vi "XYStage_Load_Command_Array.vi"(8 "error in (no error)":errorcluster, 10 "Command Enumerations":T2(ring), 11 "XY Stage Command Directory":path) -> (0 "error out":errorcluster, 2 "Enumeration Error":bool, 3 "Command Array":T1(array[cluster])=[[{"Serial Command"="ACCEL", "Expected Reply"="null"}, {"Serial Command"="AALIGN", "Expected Reply"=":A"}, {"Serial Command"="AHOME", "Expected Reply"="null"}, {"Serial Command"="AIJ", "Expected Reply"="null"}, {"Serial Command"="ARRAY", "Expected Reply"="null"}, {"Serial Command"="AZERO", "Expected Reply"="null"}, {"Serial Command"="BACKLASH", "Expected Reply"=":A"}, {"Serial Command"="BCUSTOM", "Expected Reply"="null"}, {"Serial Command"="BENABLE", "Expected Reply"="null"}, {"Serial Command"="BUILD", "Expected Reply"="null"}, {"Serial Command"="CDATE", "Expected Reply"="null"}, {"Serial Command"="CNTS", "Expected Reply"=":A"}, {"Serial Command"="CUSTOMA", "Expected Reply"="null"}, {"Serial Command"="CUSTOMB", "Expected Reply"="null"}, {"Serial Command"="DACK", "Expected Reply"=":A"}, {"Serial Command"="DUMP", "Expected Reply"="null"}, {"Serial Command"="ENSYNC", "Expected Reply"="null"}, {"Serial Command"="EPOLARITY", "Expected Reply"="null"}, {"Serial Command"="ERROR", "Expected Reply"=":A"}, {"Serial Command"="HALT", "Expected Reply"=":A"}, {"Serial Command"="HERE", "Expected Reply"=":A"}, {"Serial Command"="HOME", "Expected Reply"=":A"}, {"Serial Command"="INFO", "Expected Reply"="Ax"}, {"Serial Command"="JOYSTICK", "Expected Reply"=":A"}, {"Serial Command"="JSSPD", "Expected Reply"=":A"}, {"Serial Command"="KD", "Expected Reply"="null"}, {"Serial Command"="KI", "Expected Reply"="null"}, {"Serial Command"="KP", "Expected Reply"="null"}, {"Serial Command"="LCD", "Expected Reply"="null"}, {"Serial Command"="LED", "Expected Reply"="null"}, {"Serial Command"="LLADDR", "Expected Reply"="null"}, {"Serial Command"="LOAD", "Expected Reply"="null"}, {"Serial Command"="MAINTAIN", "Expected Reply"=":A"}, {"Serial Command"="MOTCTRL", "Expected Reply"=":A"}, {"Serial Command"="MOVE", "Expected Reply"=":A"}, {"Serial Command"="MOVREL", "Expected Reply"=":A"}, {"Serial Command"="PCROS", "Expected Reply"=":A"}, {"Serial Command"="PEDAL", "Expected Reply"=":A"}, {"Serial Command"="RBMODE", "Expected Reply"="null"}, {"Serial Command"="RDADC", "Expected Reply"=":A"}, {"Serial Command"="RDSBYTE", "Expected Reply"="null"}, {"Serial Command"="RDSTAT", "Expected Reply"=":A"}, {"Serial Command"="RESET", "Expected Reply"=":A"}, {"Serial Command"="RT", "Expected Reply"=":A"}, {"Serial Command"="RUNAWAY", "Expected Reply"=":A"}, {"Serial Command"="SAVESET", "Expected Reply"=":A"}, {"Serial Command"="SAVEPOS", "Expected Reply"=":A"}, {"Serial Command"="SCAN", "Expected Reply"="null"}, {"Serial Command"="SCANR", "Expected Reply"="null"}, {"Serial Command"="SCANV", "Expected Reply"="null"}, {"Serial Command"="SECURE", "Expected Reply"=":A"}, {"Serial Command"="SETHOME", "Expected Reply"=":A"}, {"Serial Command"="SETLOW", "Expected Reply"=":A"}, {"Serial Command"="SETUP", "Expected Reply"="null"}, {"Serial Command"="SI", "Expected Reply"=":A"}, {"Serial Command"="SPEED", "Expected Reply"=":A"}, {"Serial Command"="SPIN", "Expected Reply"=":A"}, {"Serial Command"="STATUS", "Expected Reply"="N"}, {"Serial Command"="STOPBITS", "Expected Reply"="null"}, {"Serial Command"="TTL", "Expected Reply"="null"}, {"Serial Command"="UM", "Expected Reply"=":A"}, {"Serial Command"="UNITS", "Expected Reply"=":A"}, {"Serial Command"="VB", "Expected Reply"="null"}, {"Serial Command"="VECTOR", "Expected Reply"=":A"}, {"Serial Command"="VERSION", "Expected Reply"=":A"}, {"Serial Command"="WAIT", "Expected Reply"=":A"}, {"Serial Command"="WHERE", "Expected Reply"=":A"}, {"Serial Command"="WHO", "Expected Reply"=":A"}, {"Serial Command"="WRDAC", "Expected Reply"=":A"}, {"Serial Command"="ZERO", "Expected Reply"=":A"}, {"Serial Command"="Z2B", "Expected Reply"=":A"}, {"Serial Command"="ZS", "Expected Reply"=":A"}, {"Serial Command"="OPEN", "Expected Reply"="null"}, {"Serial Command"="CLOSE", "Expected Reply"="null"}, {"Serial Command"="-0.1", "Expected Reply"="null"}, {"Serial Command"="0.1", "Expected Reply"="null"}, {"Serial Command"="75000", "Expected Reply"="null"}], [{"Serial Command"="ACCEL", "Expected Reply"="null"}, {"Serial Command"="AALIGN", "Expected Reply"=":A"}, {"Serial Command"="AHOME", "Expected Reply"="null"}, {"Serial Command"="AIJ", "Expected Reply"="null"}, {"Serial Command"="ARRAY", "Expected Reply"="null"}, {"Serial Command"="AZERO", "Expected Reply"="null"}, {"Serial Command"="BACKLASH", "Expected Reply"=":A"}, {"Serial Command"="BCUSTOM", "Expected Reply"="null"}, {"Serial Command"="BENABLE", "Expected Reply"="null"}, {"Serial Command"="BUILD", "Expected Reply"="null"}, {"Serial Command"="CDATE", "Expected Reply"="null"}, {"Serial Command"="CNTS", "Expected Reply"=":A"}, {"Serial Command"="CUSTOMA", "Expected Reply"="null"}, {"Serial Command"="CUSTOMB", "Expected Reply"="null"}, {"Serial Command"="DACK", "Expected Reply"=":A"}, {"Serial Command"="DUMP", "Expected Reply"="null"}, {"Serial Command"="ENSYNC", "Expected Reply"="null"}, {"Serial Command"="EPOLARITY", "Expected Reply"="null"}, {"Serial Command"="ERROR", "Expected Reply"=":A"}, {"Serial Command"="HALT", "Expected Reply"=":A"}, {"Serial Command"="HERE", "Expected Reply"=":A"}, {"Serial Command"="HOME", "Expected Reply"=":A"}, {"Serial Command"="INFO", "Expected Reply"="Ax"}, {"Serial Command"="JOYSTICK", "Expected Reply"=":A"}, {"Serial Command"="JSSPD", "Expected Reply"=":A"}, {"Serial Command"="KD", "Expected Reply"="null"}, {"Serial Command"="KI", "Expected Reply"="null"}, {"Serial Command"="KP", "Expected Reply"="null"}, {"Serial Command"="LCD", "Expected Reply"="null"}, {"Serial Command"="LED", "Expected Reply"="null"}, {"Serial Command"="LLADDR", "Expected Reply"="null"}, {"Serial Command"="LOAD", "Expected Reply"="null"}, {"Serial Command"="MAINTAIN", "Expected Reply"=":A"}, {"Serial Command"="MOTCTRL", "Expected Reply"=":A"}, {"Serial Command"="MOVE", "Expected Reply"=":A"}, {"Serial Command"="MOVREL", "Expected Reply"=":A"}, {"Serial Command"="PCROS", "Expected Reply"=":A"}, {"Serial Command"="PEDAL", "Expected Reply"=":A"}, {"Serial Command"="RBMODE", "Expected Reply"="null"}, {"Serial Command"="RDADC", "Expected Reply"=":A"}, {"Serial Command"="RDSBYTE", "Expected Reply"="null"}, {"Serial Command"="RDSTAT", "Expected Reply"=":A"}, {"Serial Command"="RESET", "Expected Reply"=":A"}, {"Serial Command"="RT", "Expected Reply"=":A"}, {"Serial Command"="RUNAWAY", "Expected Reply"=":A"}, {"Serial Command"="SAVESET", "Expected Reply"=":A"}, {"Serial Command"="SAVEPOS", "Expected Reply"=":A"}, {"Serial Command"="SCAN", "Expected Reply"="null"}, {"Serial Command"="SCANR", "Expected Reply"="null"}, {"Serial Command"="SCANV", "Expected Reply"="null"}, {"Serial Command"="SECURE", "Expected Reply"=":A"}, {"Serial Command"="SETHOME", "Expected Reply"=":A"}, {"Serial Command"="SETLOW", "Expected Reply"=":A"}, {"Serial Command"="SETUP", "Expected Reply"="null"}, {"Serial Command"="SI", "Expected Reply"=":A"}, {"Serial Command"="SPEED", "Expected Reply"=":A"}, {"Serial Command"="SPIN", "Expected Reply"=":A"}, {"Serial Command"="STATUS", "Expected Reply"="N"}, {"Serial Command"="STOPBITS", "Expected Reply"="null"}, {"Serial Command"="TTL", "Expected Reply"="null"}, {"Serial Command"="UM", "Expected Reply"=":A"}, {"Serial Command"="UNITS", "Expected Reply"=":A"}, {"Serial Command"="VB", "Expected Reply"="null"}, {"Serial Command"="VECTOR", "Expected Reply"=":A"}, {"Serial Command"="VERSION", "Expected Reply"=":A"}, {"Serial Command"="WAIT", "Expected Reply"=":A"}, {"Serial Command"="WHERE", "Expected Reply"=":A"}, {"Serial Command"="WHO", "Expected Reply"=":A"}, {"Serial Command"="WRDAC", "Expected Reply"=":A"}, {"Serial Command"="ZERO", "Expected Reply"=":A"}, {"Serial Command"="Z2B", "Expected Reply"=":A"}, {"Serial Command"="ZS", "Expected Reply"=":A"}, {"Serial Command"="OPEN", "Expected Reply"="null"}, {"Serial Command"="CLOSE", "Expected Reply"="null"}, {"Serial Command"="-0.1", "Expected Reply"="null"}, {"Serial Command"="0.1", "Expected Reply"="null"}, {"Serial Command"="75000", "Expected Reply"="null"}], [{"Serial Command"="ACCEL", "Expected Reply"="null"}, {"Serial Command"="AALIGN", "Expected Reply"=":A"}, {"Serial Command"="AHOME", "Expected Reply"="null"}, {"Serial Command"="AIJ", "Expected Reply"="null"}, {"Serial Command"="ARRAY", "Expected Reply"="null"}, {"Serial Command"="AZERO", "Expected Reply"="null"}, {"Serial Command"="BACKLASH", "Expected Reply"=":A"}, {"Serial Command"="BCUSTOM", "Expected Reply"="null"}, {"Serial Command"="BENABLE", "Expected Reply"="null"}, {"Serial Command"="BUILD", "Expected Reply"="null"}, {"Serial Command"="CDATE", "Expected Reply"="null"}, {"Serial Command"="CNTS", "Expected Reply"=":A"}, {"Serial Command"="CUSTOMA", "Expected Reply"="null"}, {"Serial Command"="CUSTOMB", "Expected Reply"="null"}, {"Serial Command"="DACK", "Expected Reply"=":A"}, {"Serial Command"="DUMP", "Expected Reply"="null"}, {"Serial Command"="ENSYNC", "Expected Reply"="null"}, {"Serial Command"="EPOLARITY", "Expected Reply"="null"}, {"Serial Command"="ERROR", "Expected Reply"=":A"}, {"Serial Command"="HALT", "Expected Reply"=":A"}, {"Serial Command"="HERE", "Expected Reply"=":A"}, {"Serial Command"="HOME", "Expected Reply"=":A"}, {"Serial Command"="INFO", "Expected Reply"="Ax"}, {"Serial Command"="JOYSTICK", "Expected Reply"=":A"}, {"Serial Command"="JSSPD", "Expected Reply"=":A"}, {"Serial Command"="KD", "Expected Reply"="null"}, {"Serial Command"="KI", "Expected Reply"="null"}, {"Serial Command"="KP", "Expected Reply"="null"}, {"Serial Command"="LCD", "Expected Reply"="null"}, {"Serial Command"="LED", "Expected Reply"="null"}, {"Serial Command"="LLADDR", "Expected Reply"="null"}, {"Serial Command"="LOAD", "Expected Reply"="null"}, {"Serial Command"="MAINTAIN", "Expected Reply"=":A"}, {"Serial Command"="MOTCTRL", "Expected Reply"=":A"}, {"Serial Command"="MOVE", "Expected Reply"=":A"}, {"Serial Command"="MOVREL", "Expected Reply"=":A"}, {"Serial Command"="PCROS", "Expected Reply"=":A"}, {"Serial Command"="PEDAL", "Expected Reply"=":A"}, {"Serial Command"="RBMODE", "Expected Reply"="null"}, {"Serial Command"="RDADC", "Expected Reply"=":A"}, {"Serial Command"="RDSBYTE", "Expected Reply"="null"}, {"Serial Command"="RDSTAT", "Expected Reply"=":A"}, {"Serial Command"="RESET", "Expected Reply"=":A"}, {"Serial Command"="RT", "Expected Reply"=":A"}, {"Serial Command"="RUNAWAY", "Expected Reply"=":A"}, {"Serial Command"="SAVESET", "Expected Reply"=":A"}, {"Serial Command"="SAVEPOS", "Expected Reply"=":A"}, {"Serial Command"="SCAN", "Expected Reply"="null"}, {"Serial Command"="SCANR", "Expected Reply"="null"}, {"Serial Command"="SCANV", "Expected Reply"="null"}, {"Serial Command"="SECURE", "Expected Reply"=":A"}, {"Serial Command"="SETHOME", "Expected Reply"=":A"}, {"Serial Command"="SETLOW", "Expected Reply"=":A"}, {"Serial Command"="SETUP", "Expected Reply"="null"}, {"Serial Command"="SI", "Expected Reply"=":A"}, {"Serial Command"="SPEED", "Expected Reply"=":A"}, {"Serial Command"="SPIN", "Expected Reply"=":A"}, {"Serial Command"="STATUS", "Expected Reply"="N"}, {"Serial Command"="STOPBITS", "Expected Reply"="null"}, {"Serial Command"="TTL", "Expected Reply"="null"}, {"Serial Command"="UM", "Expected Reply"=":A"}, {"Serial Command"="UNITS", "Expected Reply"=":A"}, {"Serial Command"="VB", "Expected Reply"="null"}, {"Serial Command"="VECTOR", "Expected Reply"=":A"}, {"Serial Command"="VERSION", "Expected Reply"=":A"}, {"Serial Command"="WAIT", "Expected Reply"=":A"}, {"Serial Command"="WHERE", "Expected Reply"=":A"}, {"Serial Command"="WHO", "Expected Reply"=":A"}, {"Serial Command"="WRDAC", "Expected Reply"=":A"}, {"Serial Command"="ZERO", "Expected Reply"=":A"}, {"Serial Command"="Z2B", "Expected Reply"=":A"}, {"Serial Command"="ZS", "Expected Reply"=":A"}, {"Serial Command"="OPEN", "Expected Reply"="null"}, {"Serial Command"="CLOSE", "Expected Reply"="null"}, {"Serial Command"="-0.1", "Expected Reply"="null"}, {"Serial Command"="0.1", "Expected Reply"="null"}, {"Serial Command"="75000", "Expected Reply"="null"}]])   [LabVIEW 2013]
uses:
  <vilib>/Utility/file.llb/Read From Spreadsheet File (string).vi
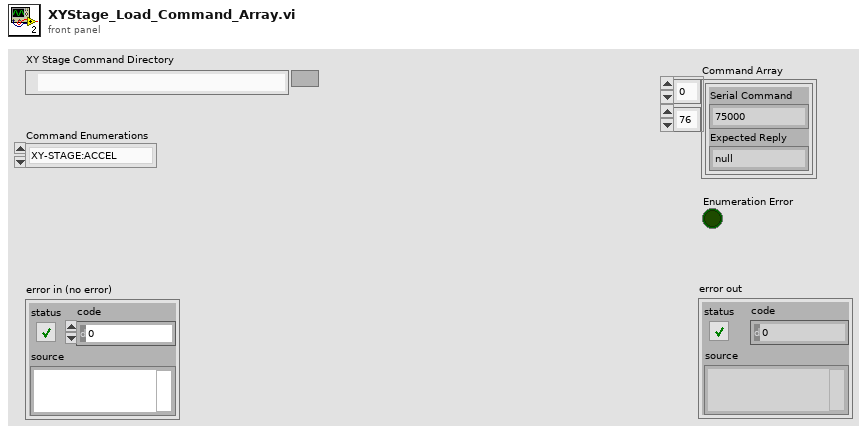
[diagram p1: front panel]
types:
  T1 = cluster{"Serial Command":string, "Expected Reply":string}[][]
  T2 = enum16{"XY-STAGE:ACCEL", "XY-STAGE:AALIGN", "XY-STAGE:AHOME", "XY-STAGE:AIJ", "XY-STAGE:ARRAY", "XY-STAGE:AZERO", "XY-STAGE:BACKLASH", "XY-STAGE:BCUSTOM", "XY-STAGE:BENABLE", "XY-STAGE:BUILD", "XY-STAGE:CDATE", "XY-STAGE:CNTS", "XY-STAGE:CUSTOMA", "XY-STAGE:CUSTOMB", "XY-STAGE:DACK", "XY-STAGE:DUMP", "XY-STAGE:ENSYNC", "XY-STAGE:EPOLARITY", "XY-STAGE:ERROR", "XY-STAGE:HALT", "XY-STAGE:HERE", "XY-STAGE:HOME", "XY-STAGE:INFO", "XY-STAGE:JOYSTICK", "XY-STAGE:JSSPD", "XY-STAGE:KD", "XY-STAGE:KI", "XY-STAGE:KP", "XY-STAGE:LCD", "XY-STAGE:LED", "XY-STAGE:LLADDR", "XY-STAGE:LOAD", "XY-STAGE:MAINTAIN", "XY-STAGE:MOTCTRL", "XY-STAGE:MOVE", "XY-STAGE:MOVREL", "XY-STAGE:PCROS", "XY-STAGE:PEDAL", "XY-STAGE:RBMODE", "XY-STAGE:RDADC", "XY-STAGE:RDSBYTE", "XY-STAGE:RDSTAT", "XY-STAGE:RESET", "XY-STAGE:RT", "XY-STAGE:RUNAWAY", "XY-STAGE:SAVESET", "XY-STAGE:SAVEPOS", "XY-STAGE:SCAN", "XY-STAGE:SCANR", "XY-STAGE:SCANV", "XY-STAGE:SECURE", "XY-STAGE:SETHOME", "XY-STAGE:SETLOW", "XY-STAGE:SETUP", "XY-STAGE:SI", "XY-STAGE:SPEED", "XY-STAGE:SPIN", "XY-STAGE:STATUS", "XY-STAGE:STOPBITS", "XY-STAGE:TTL", "XY-STAGE:UM", "XY-STAGE:UNITS", "XY-STAGE:VB", "XY-STAGE:VECTOR", "XY-STAGE:VERSION", "XY-STAGE:WAIT", "XY-STAGE:WHERE", "XY-STAGE:WHO", "XY-STAGE:WRDAC", "XY-STAGE:ZERO", "XY-STAGE:Z2B", "XY-STAGE:ZS", "XY-STAGE:OPEN", "XY-STAGE:CLOSE", "XY-STAGE:XMICRON", "XY-STAGE:YMICRON", "XY-STAGE:SPEED_MAX"}
  T3 = cluster{"Serial Command":string, "Expected Reply":string}
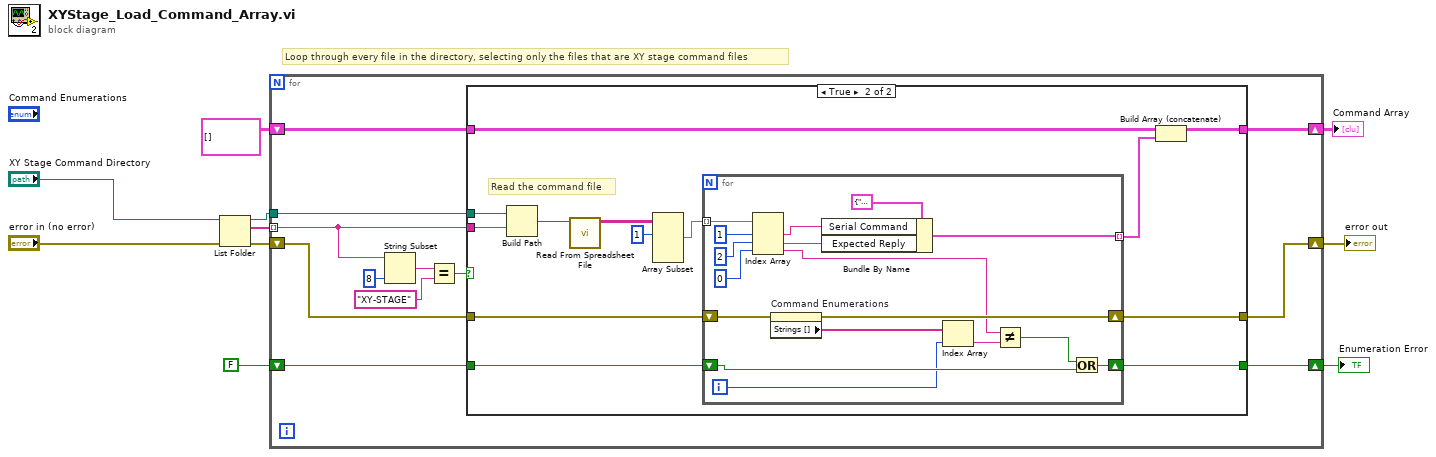
[diagram p0: block diagram]
diagram:
  # "Loop through every file in the directory, selecting only the files that are XY stage command files"
  n1 = List Folder(path="XY Stage Command Directory", error in="error in (no error)") -> (path out=w6:path, filenames=w8:string[], error out=w7:errorcluster)  [unwired: 2 in, 1 out]
  n2 = for {
    tunnel: w8 -> [w16] mode=indexing
    shift-right: [w17] -> w2
    shift-left: w7 -> [w18]
    tunnel: w6 -> [w15]
    shift-right: [w13] -> w5
    shift-left: T1 [] -> [w14]
    shift-right: [w11] -> w3
    shift-left: FALSE -> [w12]
    n3 = String Subset(string=w16, length (rest)=8 ("length (rest)")) -> (substring=w21:string)  [unwired: 1 in]
    n4 = Equal?(x=w21, y="XY-STAGE") -> (x = y?=w19:bool)
    n5 = case shown="True" w19 {
      tunnel: w18 -> [w25 w32]
      tunnel: [w25 w31] -> w17
      tunnel: w16 -> [_ w37]
      tunnel: w15 -> [_ w38]
      tunnel: w14 -> [w24 w30]
      tunnel: [w24 w29] -> w13
      tunnel: w12 -> [w23 w27]
      tunnel: [w23 w26] -> w11
      frame False {
        # "Not an XY stage command file."
      }
      frame True {
        # "Read the command file"
        n6 = Build Path(base path=w38, name or relative path=w37) -> (appended path=w36:path)
        n7 = call-poly <vilib>:"Read From Spreadsheet File.vi"("file path (dialog if empty)"=w36) -> ("all rows"=w35:string[][])  [unwired: 6 in, 4 out]
        n8 = Array Subset(array=w35, index (row)=1 ("index")) -> (w33:string[][])  [unwired: 3 in]
        n9 = for {
          tunnel: w33 -> [w55] mode=indexing
          shift-right: [w46] -> w31
          shift-left: w32 -> [w48]
          tunnel: [w43] -> w28 mode=indexing
          shift-right: [w42] -> w26
          shift-left: w27 -> [w40]
          i -> [w39]
          n10 = Index Array(array=w55, index #1=1 ("index"), index #2=2 ("index"), index #3=0 ("index")) -> (element #1=w51:string, element #2=w50:string, element #3=w44:string)
          n11 = property on="Command Enumerations" class="Enum (strict)"(error in=w48) -> (error out=w46:errorcluster, "Strings []"=w47:string[])  [unwired: 1 in, 1 out]
          n12 = Bundle By Name(cluster=T3 {"Serial Command"="", "Expected Reply"=""} ("Cluster"), "Serial Command"=w51, "Expected Reply"=w50) -> (w43:T3)
          n13 = Index Array(array=w47, index=w39) -> (element=w45:string)
          n14 = Not Equal?(x=w44, y=w45) -> (x != y?=w41:bool)
          n15 = Or(x=w41, y=w40) -> (x .or. y?=w42:bool)
        }
        n16 = Build Array (concatenate)(w30, w28) -> (w29:T1)
      }
    }
  }
  "error out" <- w2
  "Command Array" <- w5
  "Enumeration Error" <- w3
